vi "查询前序设备.vi"(7 "枚举":enum16{"电机装配", "ECU装配"}(ring), 11 "PRODUCT_ID":string) -> (3 "前序工位":string)   [LabVIEW 2020]
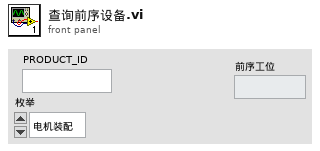
[diagram p1: front panel]
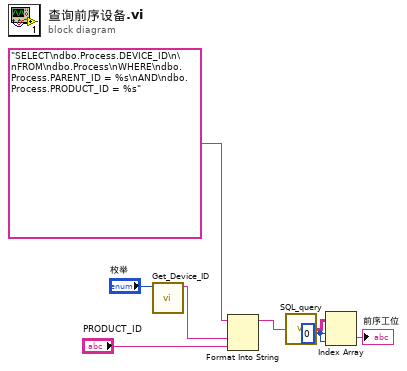
[diagram p0: block diagram]
diagram:
  w1 = 0 ("禁用的索引 (列)")
  n1 = call "Get_Device_ID.vi"("枚举"="枚举") -> ("Device_ID"=w3:string)  [unwired: 9 in, 1 out]
  n2 = Format Into String(format string="SELECT\ndbo.Process.DEVICE_ID\n\nFROM\ndbo.Process\nWHERE\ndbo.Process.PARENT_ID = %s\nAND\ndbo.Process.PRODUCT_ID = %s" ("SQL query"), w3, "PRODUCT_ID") -> (resulting string=w7:string)  [unwired: 2 in, 1 out]
  n3 = call "SQL_query.vi"("SQL query"=w7) -> ("data"=w6:string[][])  [unwired: 2 in, 2 out]
  n4 = Index Array(array=w6, index (row)=w1, index (col)=w1) -> (element=→"前序工位":string)
